vi "SetNag_record_pressure_values.vi"() -> ()   [LabVIEW 2013]
uses:
  <vilib>/Utility/file.llb/Write To Spreadsheet File (string).vi
  <vilib>/Utility/file.llb/Write To Spreadsheet File (DBL).vi
panel:
  in  "milliseconds to wait":u32=100
  in  "Write":string="_OXY\r"
  out "Read 3":string
  in  "Write 3":string="_ETA\r"
  in  "stop 2":bool
  out "Read 2":string
  in  "Write 2":string="_PAB\r"
  out "Read":string
  out "Waveform Chart":T1(graph)
  in  "Com Port":i32(ring) items=["Com 1", "Com 2", "Com 3", "Com 4", "Com 5", "Com 6", "COM 7", "COM 8", "COM 9", "COM 10", "COM 11", "COM 12", "com 13", "COM 14"]
  in  "Baud Rate":i32(ring)=2 items=["2400", "4800", "9600", "19200", "38400", "57600", "115200"]
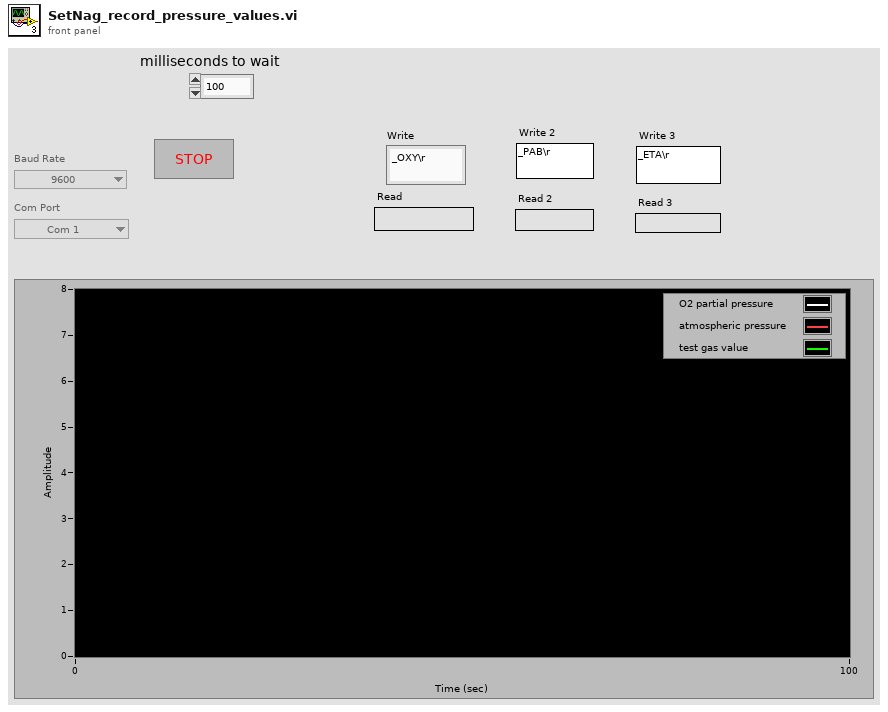
[diagram p1: front panel]
types:
  T1 = cluster{"string read":dbl, "string read":dbl, "string read":dbl}
  T2 = enum16{"no parity", "odd parity", "even parity", "mark parity", "space parity"}
  T3 = cluster{"string read":string, "string read":string, "string read":string}
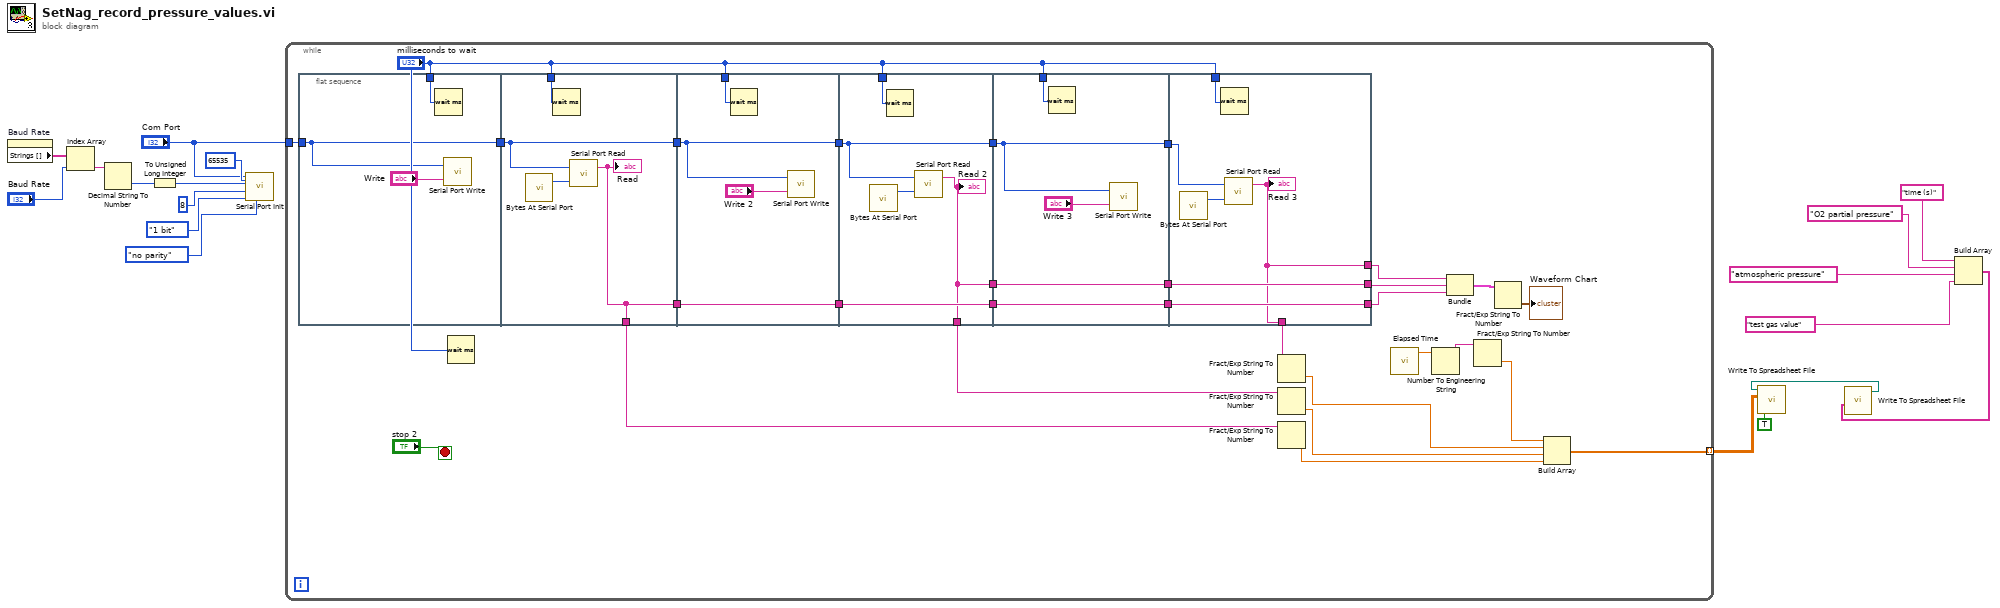
[diagram p0: block diagram]
diagram:
  n1 = property on="Baud Rate" class="Ring (strict)"() -> ("Strings []"=w17:string[])  [unwired: 2 in, 2 out]
  n2 = Index Array(array=w17, index="Baud Rate") -> (element=w16:string)
  n3 = Decimal String To Number(string=w16) -> (number=w18:i32)  [unwired: 2 in, 1 out]
  n4 = To Unsigned Long Integer(number=w18) -> (unsigned 32bit integer=w15:u32)
  n5 = call <vilib>:"Serial Port Init.vi"("parity"=T2."no parity", "buffer size"=u16 65535, "stop bits"=enum16{"1 bit", "1.5 bits", "2 bits"}."1 bit", "data bits"=u16 8, "baud rate"=w15, "port number"="Com Port") -> ()  [unwired: 1 in, 1 out]
  n6 = while {
    tunnel: "Com Port" -> [w44]
    tunnel: [w21] -> w1 mode=indexing
    stop <- "stop 2" stop-if-true
    n7 = flat-sequence {
      tunnel: w44 -> [w50]
      tunnel: [w50] -> w47
      tunnel: "milliseconds to wait" -> [w48]
      tunnel: w47 -> [w53]
      tunnel: [w53] -> w46
      tunnel: [w52] -> w38
      tunnel: [w52] -> w29
      tunnel: "milliseconds to wait" -> [w51]
      tunnel: [w57] -> w45
      tunnel: w46 -> [w57]
      tunnel: w38 -> [w56]
      tunnel: [w56] -> w37
      tunnel: "milliseconds to wait" -> [w55]
      tunnel: w45 -> [w62]
      tunnel: [w62] -> w42
      tunnel: [w60] -> w40
      tunnel: w37 -> [w61]
      tunnel: [w61] -> w36
      tunnel: [w60] -> w27
      tunnel: "milliseconds to wait" -> [w59]
      tunnel: w42 -> [w67]
      tunnel: [w67] -> w41
      tunnel: w40 -> [w66]
      tunnel: [w66] -> w39
      tunnel: w36 -> [w65]
      tunnel: [w65] -> w35
      tunnel: "milliseconds to wait" -> [w64]
      tunnel: w41 -> [w73]
      tunnel: w39 -> [w72]
      tunnel: w35 -> [w71]
      tunnel: [w70] -> w26
      tunnel: "milliseconds to wait" -> [w69]
      tunnel: [w70] -> w34
      tunnel: [w72] -> w33
      tunnel: [w71] -> w32
      frame #0 {
        n8 = Wait (ms)(milliseconds to wait=w48) -> ()  [unwired: 1 out]
        n9 = call <vilib>:"Serial Port Write.vi"("string to write"="Write", "port number"=w50) -> ()  [unwired: 1 out]
      }
      frame #1 {
        n10 = call <vilib>:"Bytes At Serial Port.vi"() -> ("byte count"=w54:u32)  [unwired: 1 in, 1 out]
        n11 = Wait (ms)(milliseconds to wait=w51) -> ()  [unwired: 1 out]
        n12 = call <vilib>:"Serial Port Read.vi"("requested byte count"=w54, "port number"=w53) -> ("string read"=w52:string)  [unwired: 1 out]
        "Read" <- w52
      }
      frame #2 {
        n13 = Wait (ms)(milliseconds to wait=w55) -> ()  [unwired: 1 out]
        n14 = call <vilib>:"Serial Port Write.vi"("string to write"="Write 2", "port number"=w57) -> ()  [unwired: 1 out]
      }
      frame #3 {
        n15 = call <vilib>:"Bytes At Serial Port.vi"() -> ("byte count"=w63:u32)  [unwired: 1 in, 1 out]
        n16 = Wait (ms)(milliseconds to wait=w59) -> ()  [unwired: 1 out]
        n17 = call <vilib>:"Serial Port Read.vi"("requested byte count"=w63, "port number"=w62) -> ("string read"=w60:string)  [unwired: 1 out]
        "Read 2" <- w60
      }
      frame #4 {
        n18 = Wait (ms)(milliseconds to wait=w64) -> ()  [unwired: 1 out]
        n19 = call <vilib>:"Serial Port Write.vi"("string to write"="Write 3", "port number"=w67) -> ()  [unwired: 1 out]
      }
      frame #5 {
        n20 = call <vilib>:"Bytes At Serial Port.vi"() -> ("byte count"=w74:u32)  [unwired: 1 in, 1 out]
        n21 = Wait (ms)(milliseconds to wait=w69) -> ()  [unwired: 1 out]
        n22 = call <vilib>:"Serial Port Read.vi"("requested byte count"=w74, "port number"=w73) -> ("string read"=w70:string)  [unwired: 1 out]
        "Read 3" <- w70
      }
    }
    n23 = Wait (ms)(milliseconds to wait="milliseconds to wait") -> ()  [unwired: 1 out]
    n24 = Fract/Exp String To Number(string=w26) -> (number=w25:dbl)  [unwired: 3 in, 1 out]
    n25 = Fract/Exp String To Number(string=w27) -> (number=w28:dbl)  [unwired: 3 in, 1 out]
    n26 = Fract/Exp String To Number(string=w29) -> (number=w24:dbl)  [unwired: 3 in, 1 out]
    n27 = call "Elapsed Time"() -> ("Elapsed Time (s)"=w23:dbl)  [unwired: 12 in, 7 out]
    n28 = Number To Engineering String(4:w23) -> (0:w22:string)  [unwired: 3 in]
    n29 = Bundle("string read"=w34, "string read"=w33, "string read"=w32) -> (w20:T3)  [unwired: 1 in]
    n30 = Fract/Exp String To Number(string=w22) -> (number=w30:dbl)  [unwired: 3 in, 1 out]
    n31 = Fract/Exp String To Number(string=w20) -> (number=→"Waveform Chart":T1)  [unwired: 3 in, 1 out]
    n32 = Build Array(w30, w25, w28, w24) -> (w21:dbl[])
  }
  n33 = Build Array("time (s)", "O2 partial pressure", "atmospheric pressure", "test gas value") -> (w6:string[])
  n34 = call-poly <vilib>:"Write To Spreadsheet File.vi"("1D data"=w6) -> ("new file path (Not A Path if cancelled)"=w8:path)  [unwired: 7 in]
  n35 = call-poly <vilib>:"Write To Spreadsheet File.vi"("append to file? (new file:F)"=TRUE, "2D data"=w1, "file path (dialog if empty)"=w8) -> ()  [unwired: 5 in, 1 out]
